vi "String Manipulation.vi"() -> ()   [LabVIEW 2014]
uses:
  <vilib>/regexp/Match Regular Expression.xnode
panel:
  out "TCP Event":bool
  out "String":string
  out "StingerVision":bool
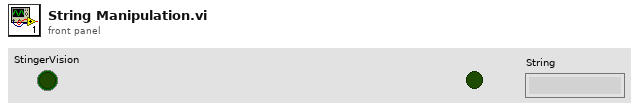
[diagram p1: front panel]
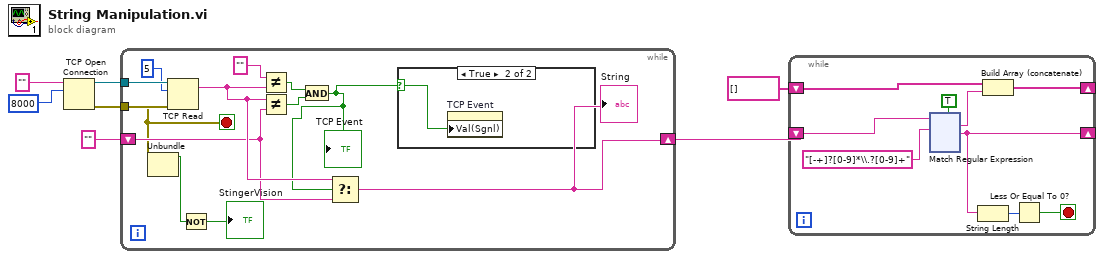
[diagram p0: block diagram]
diagram:
  n1 = TCP Open Connection(address="", remote port or service name=8000) -> (connection ID=w5:refnum<k5>, error out=w4:errorcluster)  [unwired: 3 in]
  n2 = while {
    tunnel: w5 -> [w20]
    tunnel: w4 -> [w19]
    shift-right: [w11] -> w1
    shift-left: "" -> [w13]
    stop <- w10 stop-if-true
    n3 = TCP Read(connection ID=w20, bytes to read=5, error in (no error)=w19) -> (data out=w14:string, error out=w10:errorcluster)  [unwired: 2 in, 1 out]
    n4 = Unbundle(w10) -> ("status"=w8:bool)  [unwired: 2 out]
    n5 = Not(x=w8) -> (.not. x?=→"StingerVision":bool)
    n6 = Not Equal?(x="", y=w14) -> (x != y?=w15:bool)
    n7 = Not Equal?(x=w14, y=w13) -> (x != y?=w16:bool)
    n8 = And(x=w15, y=w16) -> (x .and. y?=w12:bool)
    "TCP Event" <- w12
    n9 = Select(t=w14, s=w12, f=w13) -> (s? t:f=w11:string)
    "String" <- w11
    n10 = case shown="True" w12 {
      selector: w12 -> [_ w21]
      frame False {
      }
      frame True {
        n11 = property on="TCP Event" class="Bool (strict)"("Val(Sgnl)"=w21) -> ()  [unwired: 2 in, 2 out]
      }
    }
  }
  n12 = while {
    shift-right: [w27] -> _
    shift-left: w1 -> [w25]
    shift-right: [w23] -> _
    shift-left: string[] [] -> [w26]
    stop <- w29 stop-if-true
    n13 = xnode "Match Regular Expression"("input string"=w25, "regular expression"="[-+]?[0-9]*\\.?[0-9]+", "multiline? (F)"=TRUE) -> ("whole match"=w24:string, "after match"=w27:string)  [unwired: 3 in, 3 out]
    n14 = String Length(string=w27) -> (length=w28:i32)
    n15 = Build Array (concatenate)(w26, w24) -> (w23:string[])
    n16 = Less Or Equal To 0?(x=w28) -> (x <= 0?=w29:bool)
  }
